vi "Direction Toggle.vi"(1 "Boolean":bool) -> (0 "Boolean 2":bool)   [LabVIEW 2013]
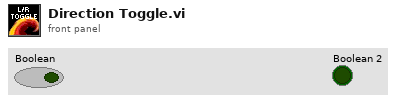
[diagram p1: front panel]
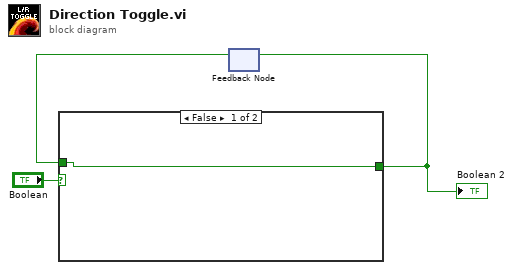
[diagram p0: block diagram]
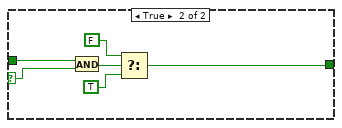
[diagram p2: hidden frame]
diagram:
  n1 = feedback #1() -> (w1:bool)  [unwired: 1 in]
  n2 = case shown="False" "Boolean" {
    selector: "Boolean" -> [_ w10]
    tunnel: w1 -> [w4 w9]
    tunnel: [w4 w5] -> w2
    frame False {
    }
    frame True {
      n3 = And(x=w9, y=w10) -> (x .and. y?=w8:bool)
      n4 = Select(t=FALSE, s=w8, f=TRUE) -> (s? t:f=w5:bool)
    }
  }
  "Boolean 2" <- w2
  n5 = feedback-in #1(w2) -> ()
